vi "Gateway.vi"() -> ()   [LabVIEW 2018]
uses:
  Gateway_States.ctl
  DataPacker/Utilities/SSH_TUNNEL.lvclass
  DataPacker/Utilities/SSH_TUNNEL.lvclass/SSH_TUNNEL.ctl
  DataPacker/DataStructures/GEM_BANK_ARRAY.lvclass
  DataPacker/DataStructures/GEM_BANK_CLUSTER_typedef.ctl
  DataPacker/DataStructures/GEM_DATA_cluster_typedef.ctl
  66a13173-cb2f-4f14-bac4-f37280f6b465.vi
  <vilib>/regexp/Match Regular Expression.xnode
panel:
  in  "Gateway IP (only needed if you have more than one network card)":string
  in  "Use Gateway to Monitor SSH traffic (recommended)":bool=TRUE
  out "Local Ports forwarded to SSH":u16[](array[numeric])
  out "MIDAS Destinations":u16[](array[numeric])
  in  "Reset open connections in memory":bool
  in  "Send Data Via SSH Tunnel":bool
  out "GEM Bank Size":i32
  in  "stop":bool
  out "Re-coded MIDAS Reply":string
  out "Forwarded ports:":i32[](array[numeric])
  out "JSON Bytes sent":i32
  out "MIDAS Forwarding Address":string
  out "error out":errorcluster
  out "bytes written":i32
  out "MIDAS Reply":string
  in  "password":string
  in  "username 2":string
  in  "ssh host port":i32=22
  in  "ssh hostname":string
  in  "MIDAS Port Number":u16
  in  "MIDAS Server (or Next Gateway)":string
  out "State":T1=enum."Send"
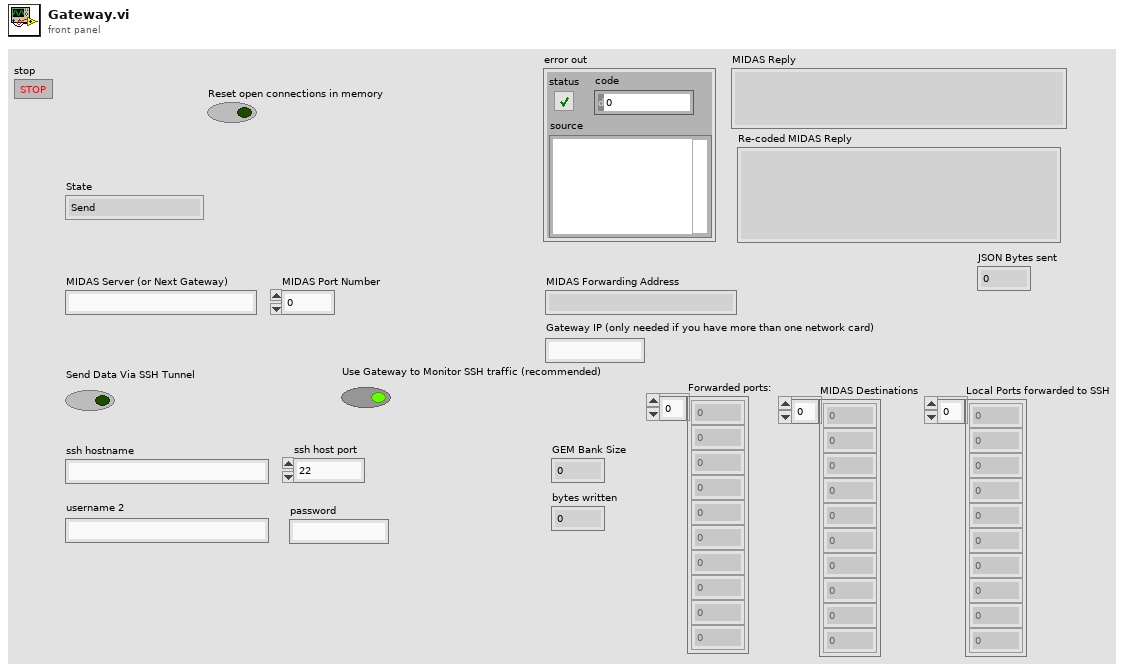
[diagram p1: front panel]
types:
  T1 = typedef "Gateway_States.ctl" = enum16{"Setup", "Connnect", "Close", "Listen", "Send", "RecodeJson", "Reply", ""}
  T2 = enum16{"big-endian, network order", "native, host order", "little-endian"}
  T3 = typedef "GEM_BANK_CLUSTER_typedef.ctl" = cluster{"Category":string, "Variable Name":string, "Equipment description":string, "History Settings":u16, "Period to update history plots":u16, "GEM_DATA Cluster":T4}
  T4 = typedef "GEM_DATA_cluster_typedef.ctl" = cluster{"DataType":string, "Formatted Data":u8[], "data byte order (Little Endian prefered)":enum16{"big-endian, network order", "native, host order", "little-endian"}}
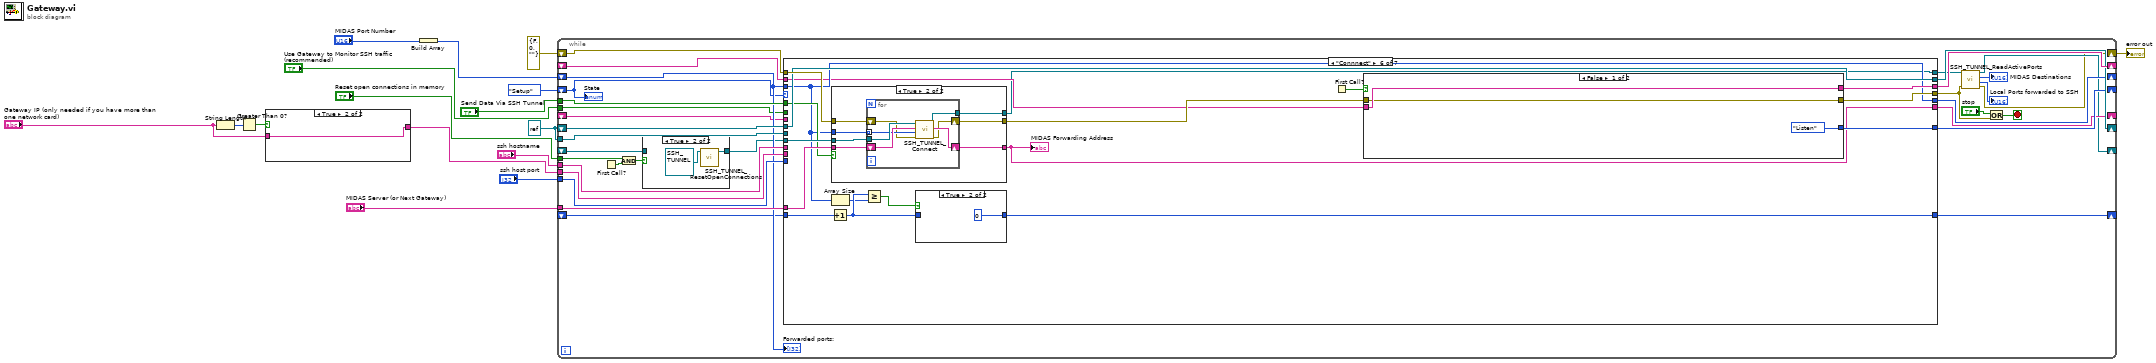
[diagram p0: block diagram]
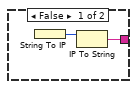
[diagram p2: hidden frame]
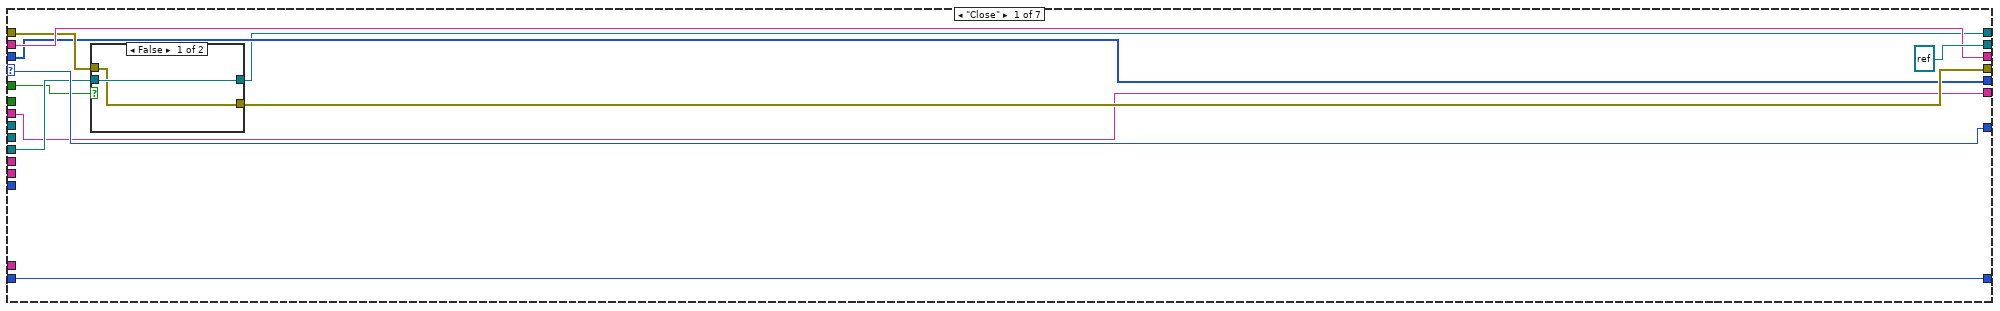
[diagram p4: hidden frame]
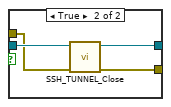
[diagram p5: hidden frame]
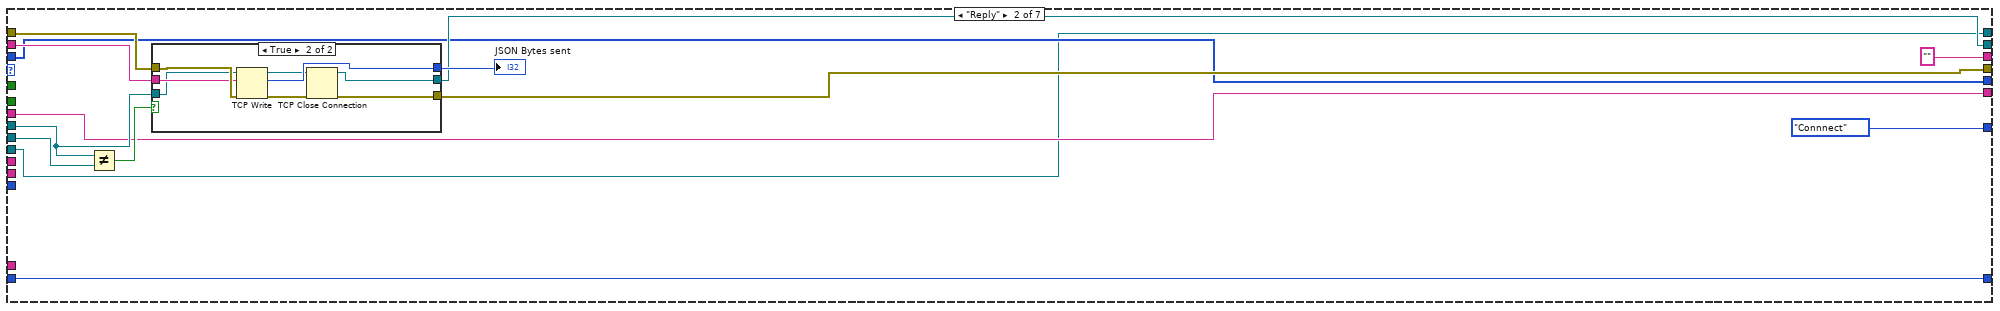
[diagram p6: hidden frame]
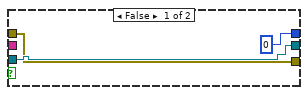
[diagram p7: hidden frame]
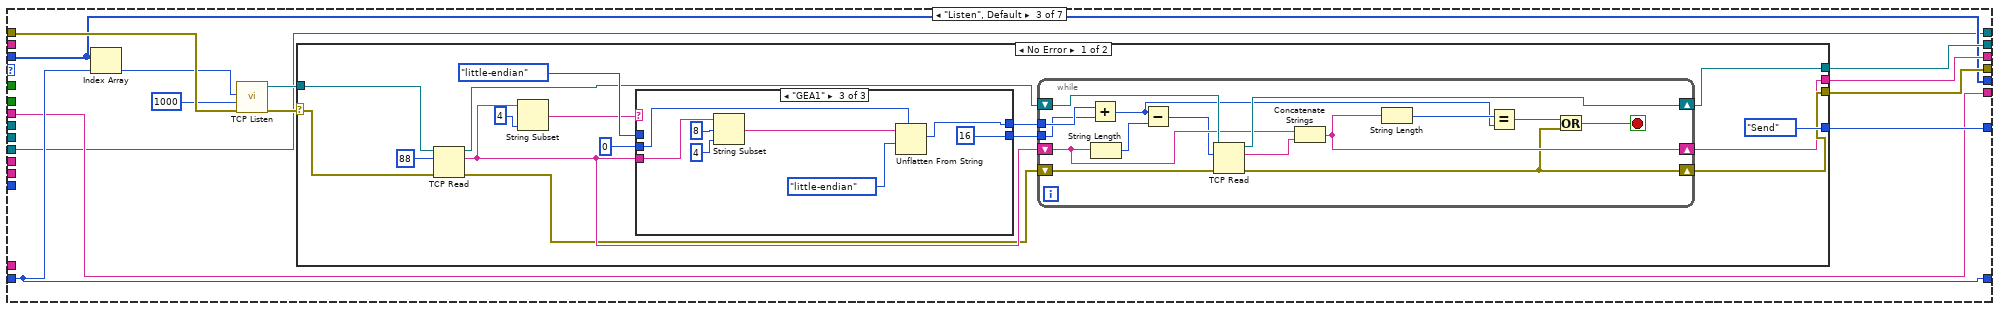
[diagram p8: hidden frame]
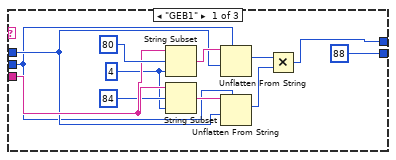
[diagram p9: hidden frame]
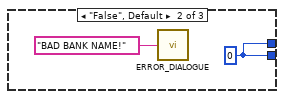
[diagram p10: hidden frame]
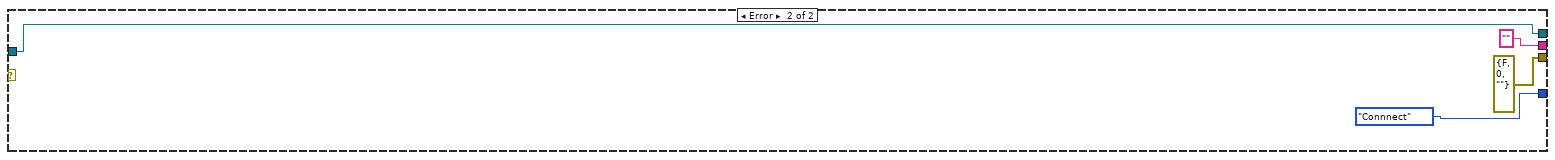
[diagram p11: hidden frame]
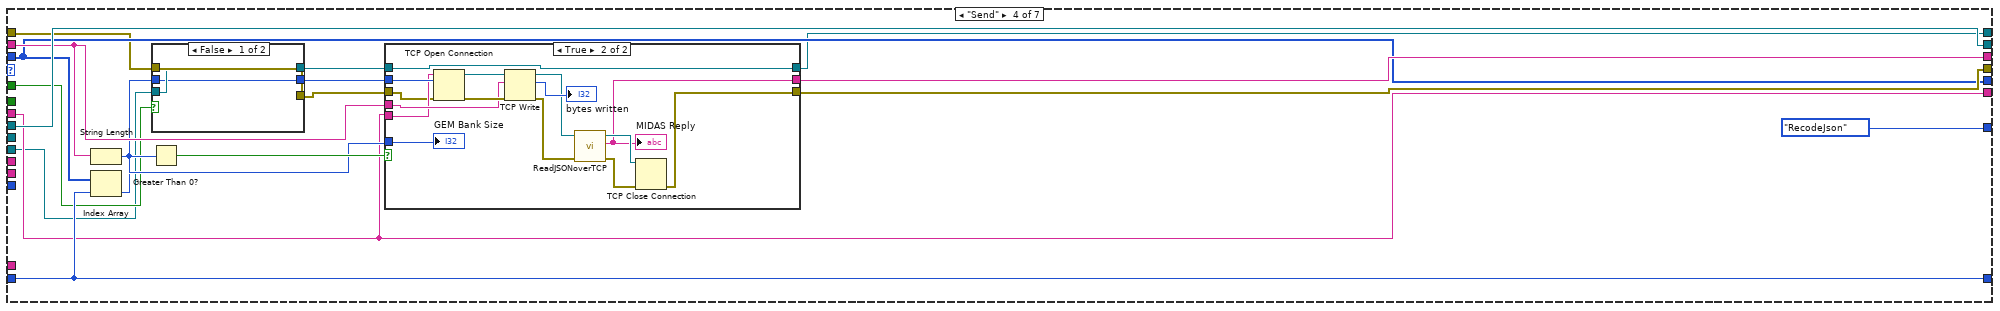
[diagram p12: hidden frame]
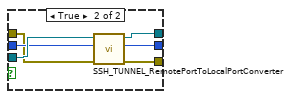
[diagram p13: hidden frame]
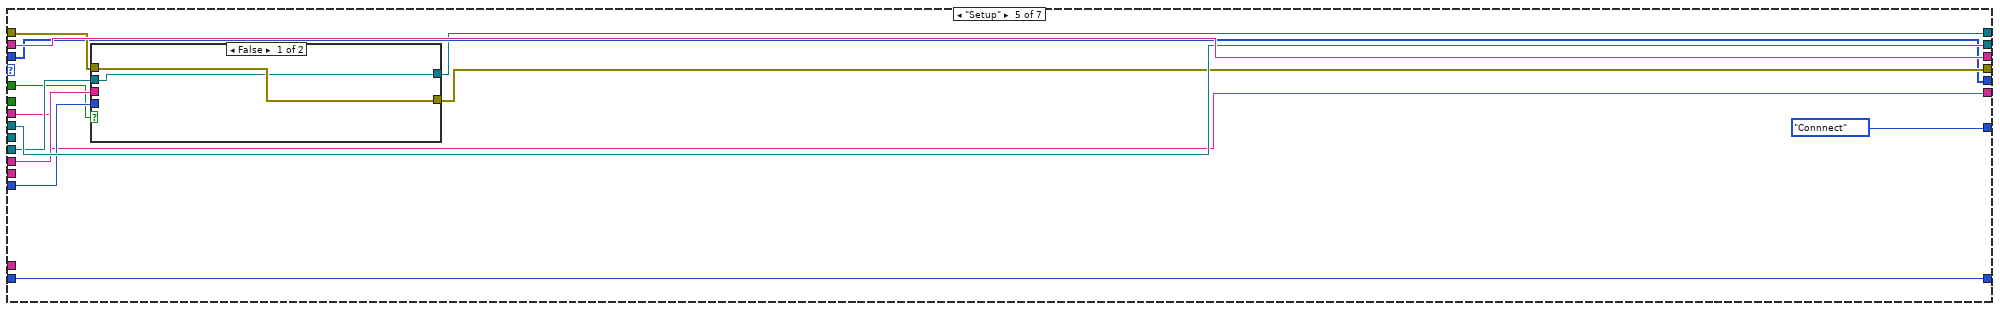
[diagram p15: hidden frame]
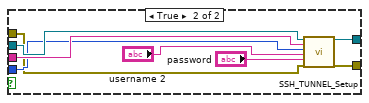
[diagram p16: hidden frame]
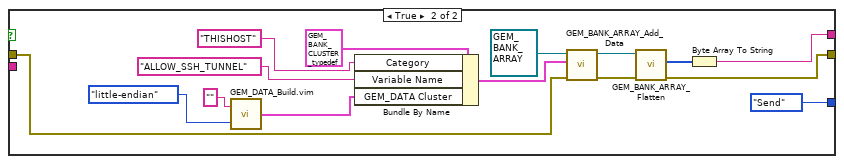
[diagram p17: hidden frame]
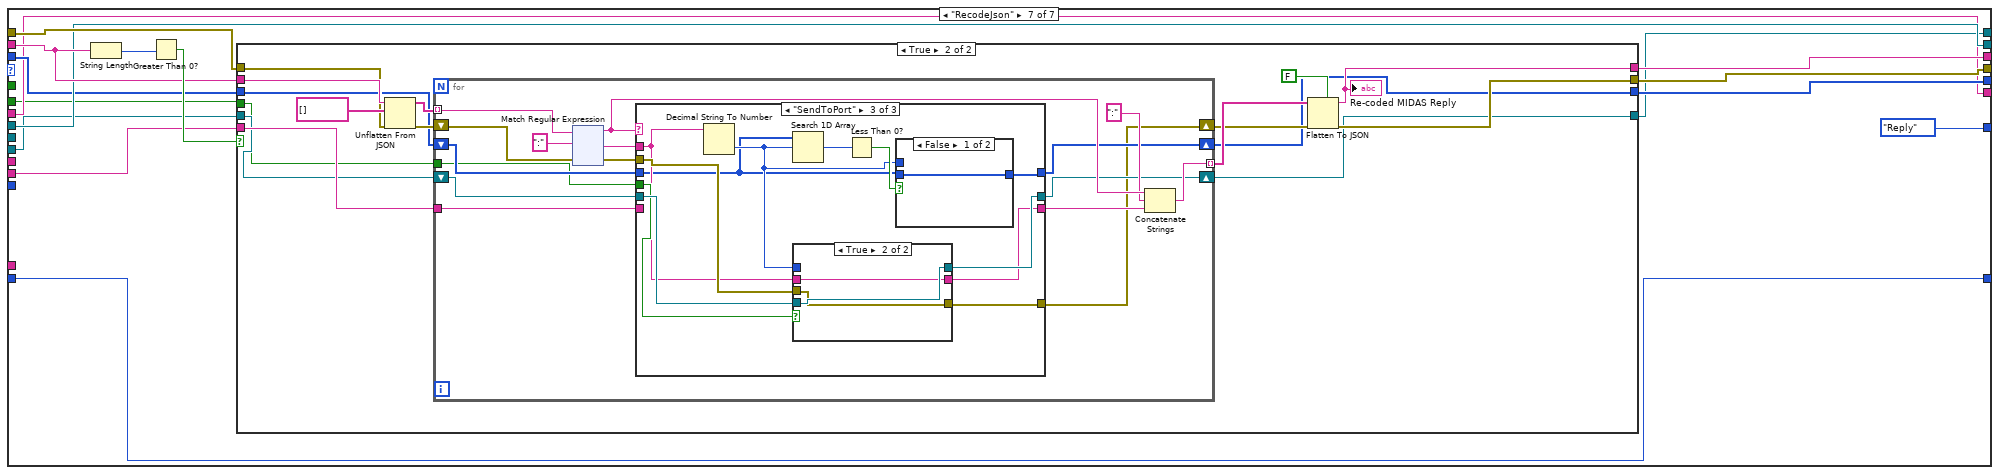
[diagram p20: hidden frame]
diagram:
  w10 = refnum<k5> refnum ("connection ID 2")
  n1 = String Length(string="Gateway IP (only needed if you have more than one network card)") -> (length=w3:i32)
  n2 = Greater Than 0?(x=w3) -> (x > 0?=w2:bool)
  n3 = case shown="True" w2 {
    tunnel: [w17 w19] -> w11
    tunnel: "Gateway IP (only needed if you have more than one network card)" -> [_ w19]
    frame False {
      n4 = String To IP() -> (0:w18:u32)  [unwired: 1 in]
      n5 = IP To String(2:w18) -> (0:w17:string)  [unwired: 1 in]
    }
    frame True {
    }
  }
  n6 = Build Array("MIDAS Port Number") -> (w8:u16[])
  n7 = while {
    shift-right: [w31] -> _
    shift-left: _ -> [w23]
    shift-right: [w27] -> w12
    shift-left: errorcluster {"status"=FALSE, "code"=0, "source"=""} ("error out") -> [w52]
    shift-right: [w47] -> _
    shift-left: Gateway_States."Setup" -> [w20]
    shift-right: [w51] -> _
    shift-left: _ -> [w48]
    shift-right: [w50] -> _
    shift-left: w10 -> [w49]
    tunnel: "MIDAS Server (or Next Gateway)" -> [w46]
    tunnel: "ssh hostname" -> [w45]
    tunnel: "ssh host port" -> [w44]
    tunnel: w11 -> [w43]
    tunnel: w10 -> [w42]
    tunnel: "Send Data Via SSH Tunnel" -> [w41]
    shift-right: [w39] -> _
    shift-left: w8 -> [w40]
    shift-right: [w37] -> _
    shift-left: _ -> [w38]
    shift-right: [w36] -> _
    shift-left: _ -> [w35]
    tunnel: "Reset open connections in memory" -> [w25]
    tunnel: "Use Gateway to Monitor SSH traffic (recommended)" -> [w21]
    stop <- w33 stop-if-true
    n8 = First Call?() -> (First Call?: T/F=w26:bool)
    n9 = And(x=w25, y=w26) -> (x .and. y?=w24:bool)
    n10 = case shown="True" w24 {
      tunnel: [w53 w55] -> w22
      tunnel: w23 -> [w53 _]
      frame False {
      }
      frame True {
        n11 = call "SSH_TUNNEL_ResetOpenConnections.vi"("SSH_TUNNEL in"=refnum<class "SSH_TUNNEL.lvclass"> refnum ("SSH_TUNNEL.lvclass")) -> ("SSH_TUNNEL out"=w55:refnum<class "SSH_TUNNEL.lvclass">)  [unwired: 9 in, 1 out]
      }
    }
    n12 = case shown="\"Connnect\"" w20 {
      selector: w20 -> [w66 _ _ _ _ _ _]
      tunnel: w22 -> [w63 w73 w98 w171 w222 w254 w294]
      tunnel: [w56 w73 w98 w175 w213 w236 w293] -> w32
      tunnel: w52 -> [w62 w82 w110 w173 w219 w252 w304]
      tunnel: [w61 w79 w107 w182 w218 w247 w303] -> w28
      tunnel: [w66 Gateway_States."Connnect" w109 Gateway_States."RecodeJson" Gateway_States."Connnect" w251 Gateway_States."Reply"] -> w47
      tunnel: [w64 "" ("JSON string") w106 w179 w224 w249 w300] -> w51
      tunnel: [refnum<k5> refnum ("connection ID") w77 w105 w181 w223 w250 w302] -> w50
      tunnel: w49 -> [_ w80 _ w181 w223 w250 w302]
      tunnel: w48 -> [w64 w81 _ w180 w224 w238 w305]
      tunnel: w46 -> [_ _ _ _ _ w253 _]
      tunnel: w45 -> [_ _ _ _ w221 _ _]
      tunnel: w44 -> [_ _ _ _ w220 _ _]
      tunnel: w43 -> [_ _ _ _ _ _ w299]
      tunnel: w42 -> [_ w84 _ _ _ _ _]
      tunnel: w41 -> [w60 _ _ w174 w217 w246 _]
      tunnel: w40 -> [w58 w76 w104 w177 w215 w243 w298]
      tunnel: [w58 w76 w104 w177 w215 w243 w297] -> w39
      tunnel: w38 -> [w59 w75 w103 w178 w216 w244 w296]
      tunnel: [w59 w75 w103 w178 w216 w245 w296] -> w37
      tunnel: [w57 w74 w100 w176 w214 w237 w295] -> w36
      tunnel: w35 -> [w57 w74 w100 w176 w214 _ w295]
      tunnel: w21 -> [_ _ _ _ _ _ w292]
      frame "Close" {
        n13 = case shown="False" w60 {
          tunnel: w63 -> [w68 w72]
          tunnel: [w68 w71] -> w56
          tunnel: w62 -> [w67 w70]
          tunnel: [w67 w69] -> w61
          frame False {
          }
          frame True {
            n14 = call "SSH_TUNNEL_Close.vi"("error in (no error)"=w70, "SSH_TUNNEL in"=w72) -> ("error out"=w69:errorcluster, "SSH_TUNNEL out"=w71:refnum<class "SSH_TUNNEL.lvclass">)  [unwired: 8 in]
          }
        }
      }
      frame "Reply" {
        n15 = Not Equal?(x=w80, y=w84) -> (x != y?=w83:bool)
        n16 = case shown="True" w83 {
          tunnel: w82 -> [w88 w97]
          tunnel: w81 -> [_ w96]
          tunnel: w80 -> [w89 w95]
          tunnel: [w88 w90] -> w79
          tunnel: [0 ("bytes written") w94] -> w78
          tunnel: [w89 w92] -> w77
          frame False {
          }
          frame True {
            n17 = TCP Write(connection ID=w95, data in=w96, error in (no error)=w97) -> (connection ID out=w93:refnum<k5>, bytes written=w94:i32, error out=w91:errorcluster)  [unwired: 1 in]
            n18 = TCP Close Connection(connection ID=w93, error in (no error)=w91) -> (connection ID out=w92:refnum<k5>, error out=w90:errorcluster)  [unwired: 1 in]
          }
        }
        "JSON Bytes sent" <- w78
      }
      frame "Listen", Default {
        n19 = Index Array(array=w104, index=w103) -> (element=w102:i32)
        n20 = call <vilib>:"TCP Listen.vi"("error in (no error)"=w110, "timeout ms (wait forever: -1)"=1000, "port"=w102) -> ("error out"=w101:errorcluster, "connection ID"=w108:refnum<k5>)  [unwired: 4 in, 3 out]
        n21 = case shown="No Error" w101 {
          selector: w101 -> [w111 _]
          tunnel: [Gateway_States."Send" Gateway_States."Connnect"] -> w109
          tunnel: w108 -> [w115 w166]
          tunnel: [w114 errorcluster {"status"=FALSE, "code"=0, "source"=""} ("error out")] -> w107
          tunnel: [w113 "" ("data out")] -> w106
          tunnel: [w112 w166] -> w105
          frame No Error {
            n22 = TCP Read(connection ID=w115, bytes to read=88, error in (no error)=w111) -> (connection ID out=w119:refnum<k5>, data out=w124:string, error out=w123:errorcluster)  [unwired: 2 in]
            n23 = String Subset(string=w124, length (rest)=4 ("length (rest)")) -> (substring=w118:string)  [unwired: 1 in]
            n24 = case shown="\"GEA1\"" w118 {
              tunnel: w124 -> [w151 _ w161]
              tunnel: u32 0 -> [w146 _ w160]
              tunnel: T2."little-endian" ("byte order (0:big-endian, network order)") -> [w147 _ _]
              tunnel: [w143 w154 w157] -> w122
              tunnel: [u32 88 ("y") w154 u32 16 ("y")] -> w125
              frame "GEB1" {
                w149 = 4 ("length (rest)")
                n25 = String Subset(string=w151, offset (0)=80, length (rest)=w149) -> (substring=w152:string)
                n26 = String Subset(string=w151, offset (0)=84, length (rest)=w149) -> (substring=w148:string)
                n27 = Unflatten From String(type=w146, binary string=w152, byte order (0:big-endian, network order)=w147) -> (value=w144:u32)  [unwired: 2 in, 2 out]
                n28 = Unflatten From String(type=w146, binary string=w148, byte order (0:big-endian, network order)=w147) -> (value=w145:u32)  [unwired: 2 in, 2 out]
                n29 = Multiply(x=w144, y=w145) -> (x*y=w143:u32)
              }
              frame "False", Default {
                w154 = u32 0
                n30 = call "ERROR_DIALOGUE.vi"("String"="BAD BANK NAME!") -> ()
              }
              frame "GEA1" {
                n31 = String Subset(string=w161, offset (0)=8, length (rest)=4 ("length (rest)")) -> (substring=w159:string)
                n32 = Unflatten From String(type=w160, binary string=w159, byte order (0:big-endian, network order)=T2."little-endian") -> (value=w157:u32)  [unwired: 2 in, 2 out]
              }
            }
            n33 = while {
              tunnel: w122 -> [w129]
              shift-right: [w139] -> w112
              shift-left: w119 -> [w141]
              shift-right: [w135] -> w113
              shift-left: w124 -> [w137]
              shift-right: [w132] -> w114
              shift-left: w123 -> [w138]
              tunnel: w125 -> [w127]
              stop <- w131 stop-if-true
              n34 = Add(x=w129, y=w127) -> (x+y=w128:u32)
              n35 = String Length(string=w137) -> (length=w130:i32)
              n36 = Subtract(x=w128, y=w130) -> (x-y=w136:u32)
              n37 = TCP Read(connection ID=w141, bytes to read=w136, error in (no error)=w138) -> (connection ID out=w139:refnum<k5>, data out=w140:string, error out=w132:errorcluster)  [unwired: 2 in]
              n38 = Concatenate Strings(w137, w140) -> (w135:string)
              n39 = String Length(string=w135) -> (length=w134:i32)
              n40 = Equal?(x=w134, y=w128) -> (x = y?=w133:bool)
              n41 = Or(x=w133, y=w132) -> (x .or. y?=w131:bool)
            }
          }
          frame Error {
          }
        }
      }
      frame "Send" {
        n42 = String Length(string=w180) -> (length=w184:i32)
        n43 = Index Array(array=w177, index=w178) -> (element=w169:i32)
        n44 = Greater Than 0?(x=w184) -> (x > 0?=w185:bool)
        n45 = case shown="False" w174 {
          tunnel: w173 -> [w188 w190]
          tunnel: [w188 w189] -> w172
          tunnel: w171 -> [w187 w194]
          tunnel: [w187 w191] -> w170
          tunnel: w169 -> [w186 w193]
          tunnel: [w186 w192] -> w168
          frame False {
          }
          frame True {
            n46 = call "SSH_TUNNEL_RemotePortToLocalPortConverter.vi"("error in (no error)"=w190, "Remote Port Number"=w193, "SSH_TUNNEL in"=w194) -> ("error out"=w189:errorcluster, "Local Port Number"=w192:u16, "SSH_TUNNEL out"=w191:refnum<class "SSH_TUNNEL.lvclass">)  [unwired: 6 in]
          }
        }
        n47 = case shown="True" w185 {
          tunnel: w170 -> [w197 w211]
          tunnel: [w197 w211] -> w175
          tunnel: w176 -> [_ w205]
          tunnel: w168 -> [_ w212]
          tunnel: w184 -> [_ w199]
          tunnel: [w195 w206] -> w182
          tunnel: w180 -> [w196 w208]
          tunnel: [w196 w200] -> w179
          tunnel: w172 -> [w195 w198]
          frame False {
          }
          frame True {
            n48 = TCP Open Connection(address=w205, remote port or service name=w212, error in (no error)=w198) -> (connection ID=w207:refnum<k5>, error out=w209:errorcluster)  [unwired: 2 in]
            n49 = TCP Write(connection ID=w207, data in=w208, error in (no error)=w209) -> (connection ID out=w204:refnum<k5>, bytes written=→"bytes written":i32, error out=w203:errorcluster)  [unwired: 1 in]
            n50 = call "ReadJSONoverTCP.vi"("error out"=w203, "connection ID"=w204) -> ("error out"=w202:errorcluster, "JSON"=w200:string, "connection ID"=w201:refnum<k5>)  [unwired: 7 in]
            "MIDAS Reply" <- w200
            n51 = TCP Close Connection(connection ID=w201, error in (no error)=w202) -> (error out=w206:errorcluster)  [unwired: 1 in, 1 out]
            "GEM Bank Size" <- w199
          }
        }
      }
      frame "Setup" {
        n52 = case shown="False" w217 {
          tunnel: w222 -> [w226 w235]
          tunnel: [w226 w234] -> w213
          tunnel: w221 -> [_ w233]
          tunnel: w220 -> [_ w232]
          tunnel: w219 -> [w227 w231]
          tunnel: [w227 w230] -> w218
          frame False {
          }
          frame True {
            n53 = call "SSH_TUNNEL_Setup.vi"("SSH_TUNNEL in"=w235, "ssh hostname"=w233, "ssh host port"=w232, "username"="username 2", "password"="password", "error in (no error)"=w231) -> ("SSH_TUNNEL out"=w234:refnum<class "SSH_TUNNEL.lvclass">, "error out"=w230:errorcluster)  [unwired: 12 in]
          }
        }
      }
      frame "Connnect" {
        n54 = case shown="True" w246 {
          tunnel: w254 -> [w276 w284]
          tunnel: w253 -> [w277 w283]
          tunnel: w243 -> [_ w282]
          tunnel: w252 -> [w275 w281]
          tunnel: [w276 w280] -> w236
          tunnel: [w277 w279] -> w237
          tunnel: [w275 w278] -> w248
          frame False {
          }
          frame True {
            n55 = for {
              tunnel: w284 -> [w291]
              tunnel: w282 -> [w289] mode=indexing
              tunnel: [w287] -> w280
              shift-right: [w286] -> w279
              shift-left: w283 -> [w290]
              shift-right: [w285] -> w278
              shift-left: w281 -> [w288]
              n56 = call "SSH_TUNNEL_Connect.vi"("error in (no error)"=w288, "MIDAS Port Number"=w289, "MIDAS Address"=w290, "SSH_TUNNEL in"=w291) -> ("error out"=w285:errorcluster, "MIDAS Address"=w286:string, "SSH_TUNNEL out"=w287:refnum<class "SSH_TUNNEL.lvclass">)  [unwired: 5 in]
            }
          }
        }
        "MIDAS Forwarding Address" <- w237
        n57 = Array Size(array=w243) -> (size(s)=w241:i32)
        n58 = Increment(x=w244) -> (x+1=w242:i32)
        n59 = Greater Or Equal?(x=w242, y=w241) -> (x >= y?=w240:bool)
        n60 = case shown="True" w240 {
          tunnel: [w273 0] -> w245
          tunnel: w242 -> [w273 _]
          frame False {
          }
          frame True {
          }
        }
        n61 = First Call?() -> (First Call?: T/F=w239:bool)
        n62 = case shown="False" w239 {
          tunnel: [Gateway_States."Listen" Gateway_States."Send"] -> w251
          tunnel: [w256 w264] -> w249
          tunnel: w248 -> [w255 w262]
          tunnel: [w255 w261] -> w247
          tunnel: w238 -> [w256 _]
          frame False {
          }
          frame True {
            n63 = call "GEM_DATA_Build.vim"("byte order (Little Endian prefered)"=T2."little-endian", "Any array in"="") -> ("GEM_BANK Cluster"=w258:T4)
            n64 = Bundle By Name(cluster=T3 {"Category"="", "Variable Name"="", "Equipment description"="", "History Settings"=0, "Period to update history plots"=0, "GEM_DATA Cluster"={"DataType"="", "Formatted Data"=[], "data byte order (Little Endian prefered)"=enum."big-endian, network order"}} ("output cluster"), "Category"="THISHOST", "Variable Name"="ALLOW_SSH_TUNNEL", "GEM_DATA Cluster"=w258) -> (w270:T3)
            n65 = call "GEM_BANK_ARRAY_Add_Data.vi"("error in (no error)"=w262, "GEM BANK Cluster"=w270, "LVBANKARRAY in"=refnum<class "GEM_BANK_ARRAY.lvclass"> refnum) -> ("error out"=w267:errorcluster, "LVBANKARRAY out"=w268:refnum<class "GEM_BANK_ARRAY.lvclass">)  [unwired: 7 in]
            n66 = call "GEM_BANK_ARRAY_Flatten.vi"("error in (no error)"=w267, "LVBANKARRAY in"=w268) -> ("error out"=w261:errorcluster, "Array"=w266:u8[])  [unwired: 7 in, 1 out]
            n67 = Byte Array To String(unsigned byte array=w266) -> (string=w264:string)
          }
        }
      }
      frame "RecodeJson" {
        n68 = String Length(string=w305) -> (length=w306:i32)
        n69 = Greater Than 0?(x=w306) -> (x > 0?=w307:bool)
        n70 = case shown="True" w307 {
          tunnel: w305 -> [w310 w324]
          tunnel: w304 -> [w311 w323]
          tunnel: [w311 w319] -> w303
          tunnel: [w310 w318] -> w300
          tunnel: w299 -> [_ w317]
          tunnel: w298 -> [w309 w316]
          tunnel: [w309 w315] -> w297
          tunnel: w294 -> [w308 w314]
          tunnel: [w308 w313] -> w293
          tunnel: w292 -> [_ w312]
          frame False {
          }
          frame True {
            n71 = Unflatten From JSON(JSON string=w324, type and defaults=string[] [] ("Array"), error in (no error)=w323) -> (value=w326:string[], error out=w325:errorcluster)  [unwired: 4 in]
            n72 = for {
              tunnel: w326 -> [w343] mode=indexing
              shift-right: [w329] -> w320
              shift-left: w325 -> [w340]
              tunnel: [w336] -> w322 mode=indexing
              tunnel: w317 -> [w335]
              shift-right: [w333] -> w315
              shift-left: w316 -> [w334]
              shift-right: [w331] -> w313
              shift-left: w314 -> [w332]
              tunnel: w312 -> [w328]
              n73 = xnode "Match Regular Expression"("input string"=w343, "regular expression"=":", "error in"=w340) -> ("before match"=w339:string, "after match"=w341:string, "error out"=w330:errorcluster)  [unwired: 3 in, 2 out]
              n74 = case shown="\"SendToPort\"" w339 {
                tunnel: w341 -> [w461 _ w471]
                tunnel: [w461 w465 w475] -> w337
                tunnel: w335 -> [_ w465 _]
                tunnel: w334 -> [w460 w464 w466]
                tunnel: [w460 w464 w467] -> w333
                tunnel: w332 -> [w458 w462 w477]
                tunnel: [w458 w462 w476] -> w331
                tunnel: w330 -> [w459 w463 w474]
                tunnel: [w459 w463 w473] -> w329
                tunnel: w328 -> [_ _ w472]
                frame "False", Default {
                }
                frame "SendToAddress" {
                }
                frame "SendToPort" {
                  n75 = Decimal String To Number(string=w471) -> (number=w468:i32)  [unwired: 2 in, 1 out]
                  n76 = Search 1D Array(1D array=w466, element=w468) -> (index of element=w470:i32)  [unwired: 1 in]
                  n77 = case shown="True" w472 {
                    tunnel: w477 -> [w488 w491]
                    tunnel: [w487 w491] -> w476
                    tunnel: w468 -> [w486 _]
                    tunnel: [w484 w490] -> w475
                    tunnel: w474 -> [w483 w489]
                    tunnel: [w482 w489] -> w473
                    tunnel: w471 -> [_ w490]
                    frame False {
                      n78 = call "SSH_TUNNEL_RemotePortToLocalPortConverter.vi"("error in (no error)"=w483, "Remote Port Number"=w486, "SSH_TUNNEL in"=w488) -> ("error out"=w482:errorcluster, "Local Port Number"=w485:u16, "SSH_TUNNEL out"=w487:refnum<class "SSH_TUNNEL.lvclass">)  [unwired: 6 in]
                      n79 = Number To Decimal String(number=w485) -> (decimal integer string=w484:string)  [unwired: 1 in]
                    }
                    frame True {
                    }
                  }
                  n80 = Less Than 0?(x=w470) -> (x < 0?=w469:bool)
                  n81 = case shown="False" w469 {
                    tunnel: w466 -> [w478 w481]
                    tunnel: w468 -> [_ w480]
                    tunnel: [w478 w479] -> w467
                    frame False {
                    }
                    frame True {
                      n82 = Build Array (concatenate)(w481, w480) -> (w479:i32[])
                    }
                  }
                }
              }
              n83 = Concatenate Strings(w339, ":" ("string"), w337) -> (w336:string)
            }
            n84 = Flatten To JSON(enable LabVIEW extensions? (T)=FALSE, anything=w322, error in (no error)=w320) -> (JSON string=w318:string, 11:w319:errorcluster)
            "Re-coded MIDAS Reply" <- w318
          }
        }
      }
    }
    n85 = call "SSH_TUNNEL_ReadActivePorts.vi"("error in (no error)"=w28, "SSH_TUNNEL in"=w32) -> ("error out"=w27:errorcluster, "Local Ports forwarded to SSH"=→"Local Ports forwarded to SSH":u16[], "MIDAS Destinations"=→"MIDAS Destinations":u16[], "SSH_TUNNEL out"=w31:refnum<class "SSH_TUNNEL.lvclass">)  [unwired: 6 in]
    n86 = Or(x="stop", y=w28) -> (x .or. y?=w33:bool)
    "State" <- w20
    "Forwarded ports:" <- w40
  }
  "error out" <- w12
